vi "Check For Nested Messages With Oneofs.vi"(11 "Message Metadata":T1[](array[typedef])) -> (3 "Message Metadata":T1[](array[typedef]))   [LabVIEW 2019, in "gRPC Template Creation Utility.lvlib"]
uses:
  gRPC Template Creation Utility.lvlib
  TypeDefs/Message Metadata (Scripting).ctl
  TypeDefs/Message Element Metadata (Scripting).ctl
  TypeDefs/Message Element Type.ctl
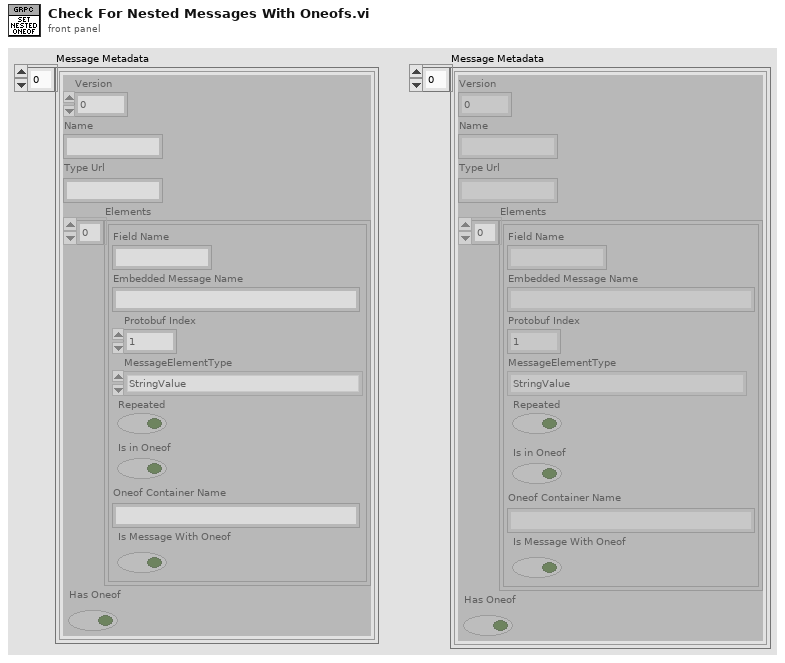
[diagram p1: front panel]
types:
  T1 = typedef "gRPC Template Creation Utility.lvlib/Message Metadata (Scripting).ctl" = cluster{"Version":i32, "Name":string, "Type Url":string, "Elements":T2[], "Has Oneof":bool}
  T2 = typedef "gRPC Template Creation Utility.lvlib/Message Element Metadata (Scripting).ctl" = cluster{"Field Name":string, "Embedded Message Name":string, "Protobuf Index":i32, "MessageElementType":T3, "Repeated":bool, "Is in Oneof":bool, "Oneof Container Name":string, "Is Message With Oneof":bool}
  T3 = typedef "gRPC Template Creation Utility.lvlib/Message Element Type.ctl" = enum32{"Int32Value", "FloatValue", "DoubleValue", "BoolValue", "StringValue", "MessageValue", "Int64Value", "UInt32Value", "UInt64Value", "EnumValue", "Bytes", "Fixed64", "Fixed32", "SFixed64", "SFixed32", "SInt64", "SInt32"}
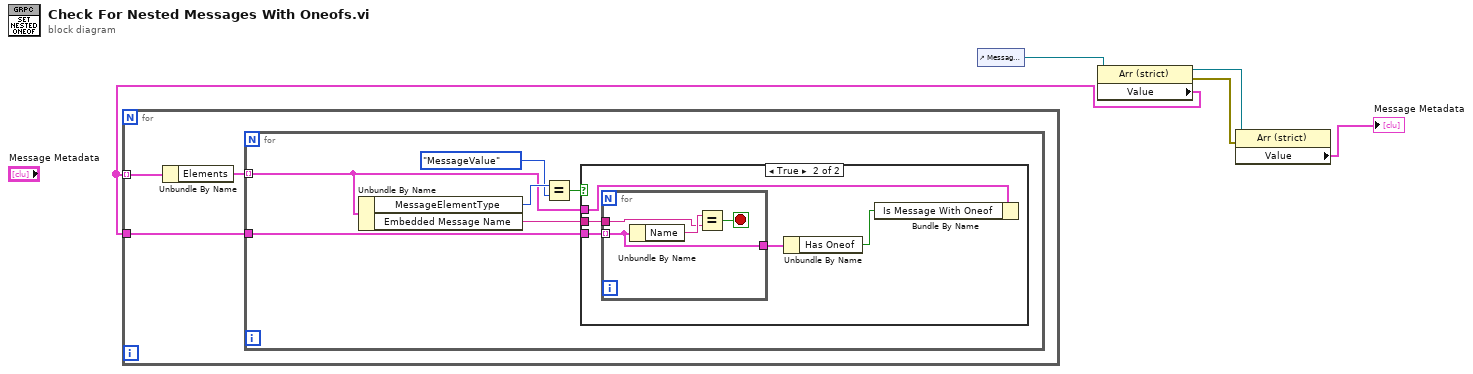
[diagram p0: block diagram]
diagram:
  n1 = control-ref of="Message Metadata"() -> (w5:refnum<vi>)
  n2 = property class="Arr (strict)"(reference=w5) -> (reference out=w1:refnum<vi>, error out=w2:errorcluster, "Value"=w4:T1[])  [unwired: 1 in]
  n3 = for {
    tunnel: w4 -> [w8] mode=indexing
    tunnel: w4 -> [w6]
    n4 = Unbundle By Name(w8) -> ("Elements"=w7:T2[])
    n5 = for {
      tunnel: w7 -> [w9] mode=indexing
      tunnel: w6 -> [w10]
      n6 = Unbundle By Name(w9) -> ("MessageElementType"=w14:T3, "Embedded Message Name"=w11:string)
      n7 = Equal?(x=w14, y=Message_Element_Type."MessageValue") -> (x = y?=w12:bool)
      n8 = case shown="True" w12 {
        tunnel: w11 -> [_ w18]
        tunnel: w10 -> [_ w19]
        tunnel: w9 -> [_ w16]
        frame False {
        }
        frame True {
          n9 = for {
            tunnel: w19 -> [w20] mode=indexing
            tunnel: w18 -> [w22]
            tunnel: [w20] -> w17
            stop <- w21 stop-if-true
            n10 = Unbundle By Name(w20) -> ("Name"=w23:string)
            n11 = Equal?(x=w23, y=w22) -> (x = y?=w21:bool)
          }
          n12 = Unbundle By Name(w17) -> ("Has Oneof"=w15:bool)
          n13 = Bundle By Name(cluster=w16, "Is Message With Oneof"=w15) -> ()  [unwired: 1 out]
        }
      }
    }
  }
  n14 = property class="Arr (strict)"(reference=w1, error in=w2) -> ("Value"=→"Message Metadata":T1[])  [unwired: 2 out]
